vi "Is Done.vi"(8 "error in (no error)":errorcluster caption="错误输入（无错误）", 11 "Iterator(Abstract) 输入":refnum<class "具体迭代器.lvclass"> caption="DNL_LabVIEW Object in") -> (0 "error out":errorcluster caption="错误输出", 1 "done":bool, 3 "Iterator(Abstract) 输出":refnum<class "具体迭代器.lvclass"> caption="DNL_LabVIEW Object out")   [LabVIEW 2011, in "迭代器.lvlib" / "具体迭代器.lvclass"]
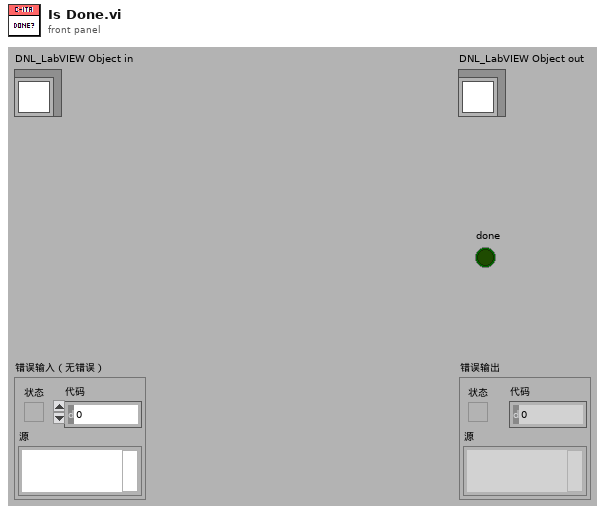
[diagram p1: front panel]
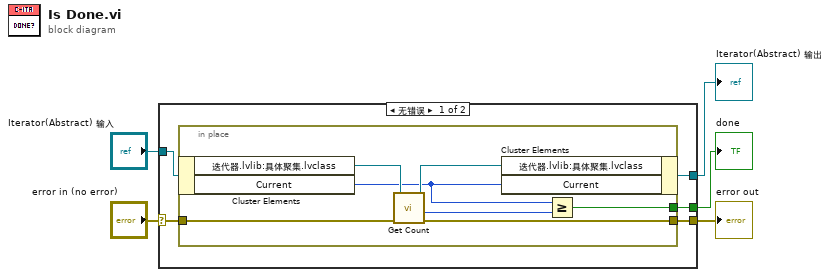
[diagram p0: block diagram]
diagram:
  n1 = case shown="无错误" "error in (no error)" {
    selector: "error in (no error)" -> [w9 w18]
    tunnel: [w8 w18] -> w4
    tunnel: "Iterator(Abstract) 输入" -> [w10 w19]
    tunnel: [w6 w19] -> w2
    tunnel: [w7 _] -> w1
    frame No Error {
      n2 = in-place {
        in-place-border: w9 -> [w15]
        in-place-border: [w14] -> w8
        in-place-border: [w12] -> w7
        n3 = in-place-cluster #1(w10) -> ("迭代器.lvlib:具体聚集.lvclass"=w17:refnum<class "具体聚集.lvclass">, "Current"=w11:i32)
        n4 = call "Get Count.vi"("error in (no error)"=w15, "具体聚集 输入"=w17) -> ("error out"=w14:errorcluster, "Count"=w13:i32, "具体聚集 输出"=w16:refnum<class "具体聚集.lvclass">)  [unwired: 7 in]
        n5 = in-place-cluster #1("迭代器.lvlib:具体聚集.lvclass"=w16, "Current"=w11) -> (w6:refnum<class "具体迭代器.lvclass">)
        n6 = Greater Or Equal?(x=w11, y=w13) -> (x >= y?=w12:bool)
      }
    }
    frame Error {
    }
  }
  "error out" <- w4
  "Iterator(Abstract) 输出" <- w2
  "done" <- w1
